vi "Result.Merge SW List Items.vi"(9 "Old Items":T1[](array[typedef]), 11 "New Items":T1[](array[typedef])) -> (3 "Merged Items":T1[](array[typedef]))   [LabVIEW 2024]
uses:
  Result XML/TestResult.SW Item.ctl
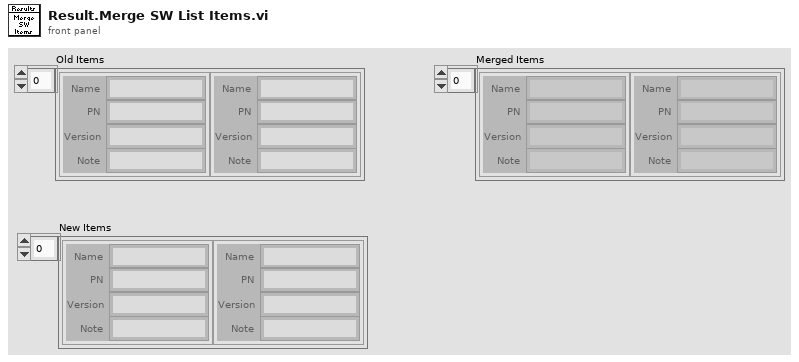
[diagram p1: front panel]
types:
  T1 = typedef "TestResult.SW Item.ctl" = cluster{"Name":string, "PN":string, "Version":string, "Note":string}
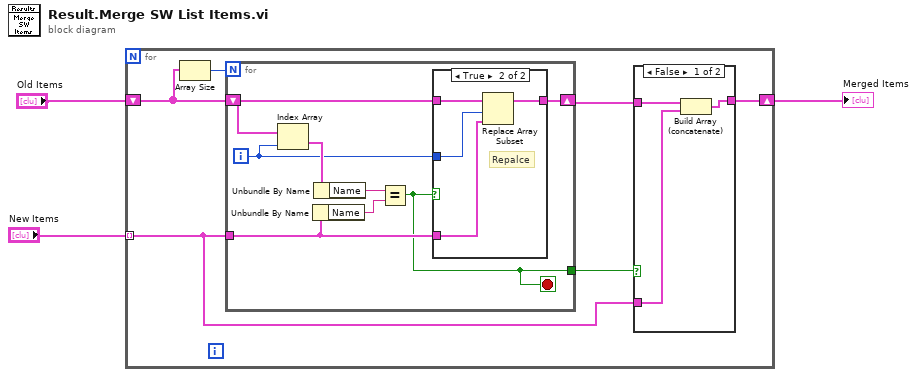
[diagram p0: block diagram]
diagram:
  n1 = for {
    tunnel: "New Items" -> [w9] mode=indexing
    shift-right: [w7] -> w1
    shift-left: "Old Items" -> [w4]
    n2 = Array Size(array=w4) -> (size(s)=w5:i32)
    n3 = for {
      N: w5 -> [_]
      tunnel: w9 -> [w19]
      tunnel: [w14] -> w6
      shift-right: [w18] -> w8
      shift-left: w4 -> [w15]
      i -> [w16]
      stop <- w14 stop-if-true
      n4 = Index Array(array=w15, index=w16) -> (element=w17:T1)
      n5 = Unbundle By Name(w19) -> ("Name"=w20:string)
      n6 = Unbundle By Name(w17) -> ("Name"=w21:string)
      n7 = Equal?(x=w21, y=w20) -> (x = y?=w14:bool)
      n8 = case shown="True" w14 {
        tunnel: w19 -> [_ w23]
        tunnel: w15 -> [w22 w26]
        tunnel: [w22 w25] -> w18
        tunnel: w16 -> [_ w24]
        frame False {
        }
        frame True {
          # "Repalce"
          n9 = Replace Array Subset(array=w26, new element=w23, index=w24) -> (w25:T1[])
        }
      }
    }
    n10 = case shown="False" w6 {
      tunnel: w9 -> [w11 _]
      tunnel: w8 -> [w12 w13]
      tunnel: [w10 w13] -> w7
      frame False {
        n11 = Build Array (concatenate)(w12, w11) -> (w10:T1[])
      }
      frame True {
      }
    }
  }
  "Merged Items" <- w1
